vi "Scan.vi"(1 "Image Resolution":u16(ring)=64 items=["32"=32, "64"=64, "128"=128, "256"=256, "1024"=1024, "2048"=2048], 2 "Scanning":bool) -> (0 "Finished?":bool)   [LabVIEW 2015]
uses:
  D:/LabVIEW for ezAFM/LV-PGC 2019-05a/Special Equipment/ezAFM/NMI Integration Code/ezCommander.dll
  LabVIEW for ezAFM/LV-PGC 2019-05a/Special Equipment/ezAFM/NMI Integration Code/ezCommander.dll
  LabVIEW for ezAFM/LV-PGC 2019-05a/Universal vi's/Global Variables/Globals-EasyAFM.vi
  Globals.vi
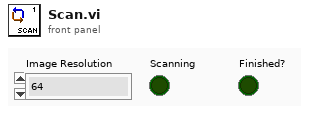
[diagram p1: front panel]
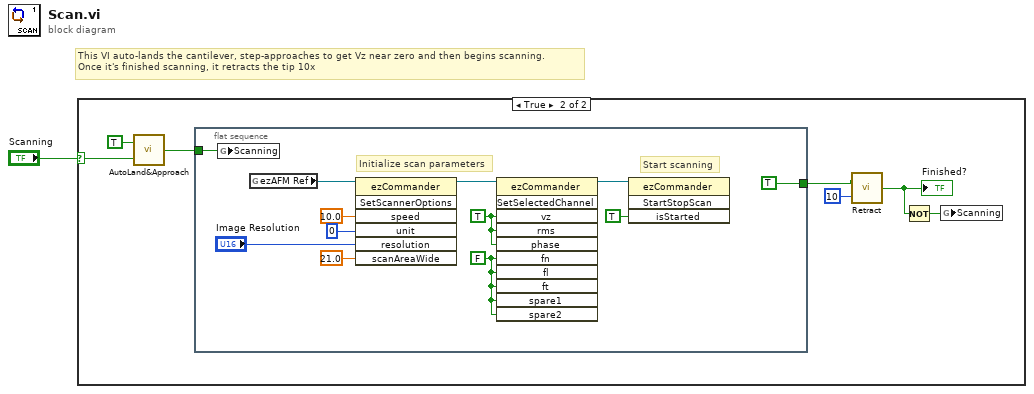
[diagram p0: block diagram]
diagram:
  # "This VI auto-lands the cantilever, step-approaches to get Vz near zero and then begins scanning.\nOnce it's finished scanning, it retracts the tip 10x"
  n1 = case shown="True" "Scanning" {
    selector: "Scanning" -> [_ w4]
    frame False {
    }
    frame True {
      n2 = call "AutoLand&Approach.vi"("Autoland?"=w4, "Step-Approach?"=TRUE) -> ("Finished?"=w3:bool)
      n3 = flat-sequence {
        tunnel: w3 -> [w20]
        tunnel: [TRUE ("Approaching?")] -> w2
        frame #0 {
          w14 = FALSE
          w15 = TRUE
          # "Initialize scan parameters"
          # "Start scanning"
          n4 = global write "Globals.vi" "Scanning"(w20) -> ()
          n5 = global read "Globals-EasyAFM.vi" "ezAFM Ref"() -> (w13:refnum<k24>)
          n6 = invoke class="ezCommander" method="SetScannerOptions"(reference=w13, "speed"=10.0, "unit"=0, "resolution"="Image Resolution", "scanAreaWide"=21.0) -> (reference out=w12:refnum<k24>)  [unwired: 2 in, 6 out]
          n7 = invoke class="ezCommander" method="SetSelectedChannel"(reference=w12, "vz"=w15, "rms"=w15, "phase"=w15, "fn"=w14, "fl"=w14, "ft"=w14, "spare1"=w14, "spare2"=w14) -> (reference out=w19:refnum<k24>)  [unwired: 2 in, 10 out]
          n8 = invoke class="ezCommander" method="StartStopScan"(reference=w19, "isStarted"=TRUE) -> ()  [unwired: 2 in, 4 out]
        }
      }
      n9 = call "Retract.vi"("Number of Cycles"=10, "Retracting?"=w2) -> ("Finished?"=w8:bool)
      "Finished?" <- w8
      n10 = Not(x=w8) -> (.not. x?=w6:bool)
      n11 = global write "Globals.vi" "Scanning"(w6) -> ()
    }
  }
